vi "Get Report Info Indexes.vi"(10 "data allocations":T1, 11 "Sequencer Module configuration in":refnum<class "Sequencer Module configuration.lvclass">) -> (0 "error out":errorcluster, 3 "Cluster":T4)   [LabVIEW 2015, in "Sequencer Module runtime.lvclass"]
uses:
  Sequencer Module runtime.lvclass
  <vilib>/NI/Tag Bus Module Framework/channel/data tables.ctl
  <vilib>/NI/Tag Bus/dictionary/data dictionary.lvclass
  <vilib>/NI/Tag Bus/dictionary table pair.ctl
  <vilib>/NI/Tag Bus/table/data table.ctl
  configuration/Sequencer Module configuration.lvclass
  <vilib>/NI/Tag Bus Module Framework/channel/TBM channel.lvclass/TBM channel.ctl
  <vilib>/NI/Tag Bus/tag/tag descriptor.lvclass/tag descriptor.ctl
  <vilib>/NI/Tag Bus/tag/read tag name.vi
  <vilib>/NI/Tag Bus/tag/read data type.vi
  <vilib>/NI/Tag Bus/dictionary/locate tag.vi
  <vilib>/NI/Tag Bus Module Framework/channel/TBM channel.lvclass
  <vilib>/NI/Tag Bus/table/data table.lvlib
  <vilib>/NI/Tag Bus/tag bus.lvlib
types:
  T1 = typedef "TBM channel.lvclass/data tables.ctl" = cluster{"input data":T2, "processing parameter":T2, "processing result":T2, "output data":T2}
  T2 = typedef "tag bus.lvlib/dictionary table pair.ctl" = cluster{"data dictionary":refnum<class "data dictionary.lvclass">, "data table":T3}
  T3 = typedef "tag bus.lvlib/data table.lvlib/data table.ctl" = cluster{"Double":dbl[], "Single":sgl[], "I64":i64[], "I32":i32[], "I16":i16[], "I8":i8[], "U64":u64[], "U32":u32[], "U16":u16[], "U8":u8[], "Boolean":bool[], "String":string[], "Array of Double":cluster{"DBL Array":dbl[]}[], "Array of Single":cluster{"SGL Array":sgl[]}[], "Array of I64":cluster{"I64 Array":i64[]}[], "Array of I32":cluster{"I32 Array":i32[]}[], "Array of I16":cluster{"I16 Array":i16[]}[], "Array of I8":cluster{"I8 Array":i8[]}[], "Array of U64":cluster{"U64 Array":u64[]}[], "Array of U32":cluster{"U32 Array":u32[]}[], "Array of U16":cluster{"U16 Array":u16[]}[], "Array of U8":cluster{"U8 Array":u8[]}[], "Array of Boolean":cluster{"Boolean Array":bool[]}[], "Array of String":cluster{"String Array":string[]}[]}
  T4 = cluster{"Station ID":i32, "Station SN":i32, "DUT SN":i32, "DUT Info":i32}
  T5 = typedef "TBM channel.lvclass/channel classification.ctl" = enum16{"input data", "output data", "processing parameter", "processing result"}
  T6 = cluster{"[0]":i32, "[1]":i32, "[2]":i32, "[3]":i32}
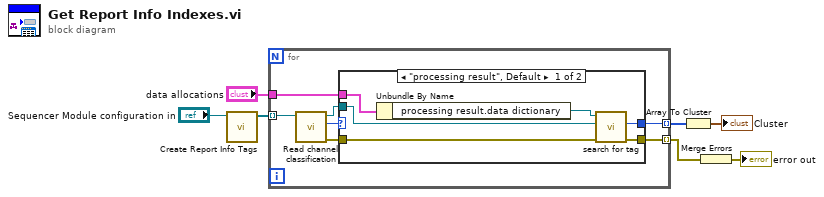
[diagram p0: block diagram]
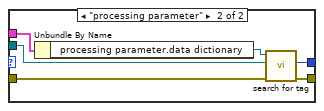
[diagram p2: hidden frame]
diagram:
  n1 = call "Create Report Info Tags.vi"("Sequencer Module configuration in"="Sequencer Module configuration in") -> ("Array"=w1:refnum<class "TBM channel.lvclass">[])  [unwired: 10 in]
  n2 = for {
    tunnel: "data allocations" -> [w11]
    tunnel: w1 -> [w10] mode=indexing
    tunnel: [w9] -> w6 mode=indexing
    tunnel: [w8] -> w4 mode=indexing
    n3 = call <vilib>:"Read channel classification.vi"("channel in"=w10) -> ("error out"=w12:errorcluster, "channel classification"=w14:T5, "channel out"=w13:refnum<class "TBM channel.lvclass">)  [unwired: 8 in]
    n4 = case shown="\"processing result\", Default" w14 {
      tunnel: w11 -> [w19 w26]
      tunnel: w13 -> [w15 w24]
      tunnel: [w18 w23] -> w9
      tunnel: w12 -> [w17 w22]
      tunnel: [w16 w21] -> w8
      frame "processing result", Default {
        n5 = Unbundle By Name(w19) -> ("processing result.data dictionary"=w20:refnum<class "data dictionary.lvclass">)
        n6 = call <vilib>:"search for tag.vi"("error in"=w17, "system tag"=w15, "data dictionary in"=w20) -> ("error out"=w16:errorcluster, "index"=w18:i32)  [unwired: 6 in, 1 out]
      }
      frame "processing parameter" {
        n7 = Unbundle By Name(w26) -> ("processing parameter.data dictionary"=w25:refnum<class "data dictionary.lvclass">)
        n8 = call <vilib>:"search for tag.vi"("error in"=w22, "system tag"=w24, "data dictionary in"=w25) -> ("error out"=w21:errorcluster, "index"=w23:i32)  [unwired: 6 in, 1 out]
      }
    }
  }
  n9 = Array To Cluster(array=w6) -> (cluster=→"Cluster":T6)
  n10 = Merge Errors(w4) -> (→"error out":errorcluster)
